vi "温度湿度监测界面.vi"() -> ()   [LabVIEW 2016, in "环境动力监测库.lvlib"]
uses:
  <vilib>/Utility/config.llb/NI_LVConfig.lvlib
  <vilib>/ptbypt/NI_PtbyPt.lvlib
panel:
  in  "湿度下限告警点":dbl
  in  "湿度上限告警点":dbl
  in  "室温下限告警点":dbl
  in  "室温上限告警点":dbl
  out "湿度":string="75.5 %"
  out "室温":string="25.8 ℃"
  # "温度湿度监测"
  # "室温:"
  # "湿度:"
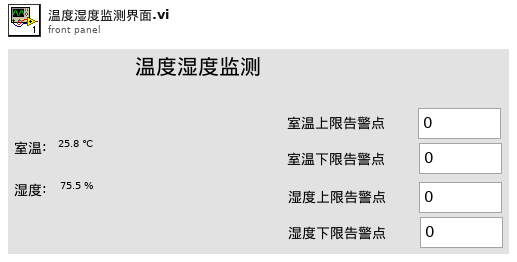
[diagram p1: front panel]
types:
  T1 = typedef "NI_LVConfig.lvlib/Config Data RefNum.ctl" = refnum<k1>
  T2 = cluster{"AD0":sgl, "AD1":sgl, "AD2":sgl, "AD3":sgl, "AD4":sgl, "AD5":sgl}
  T3 = cluster{"漏水监测配置":cluster{"监测项描述:输出":string, "端口:":enum16{"AI0", "AI1", "AI2", "AI3", "AI4", "DI0", "DI1", "DI2", "DI3", "DI4", "X0", "X1", "X2", "X3", "X4", "X5", "X6", "X7", "X8", "X9"}, "告警参数:":enum32{"禁用告警", "闭合告警", "断开告警"}, "传感器型号:":enum16{"PLC", "ZLAN"}}, "门禁开关监测配置":cluster{"监测项描述:输出":string, "端口:":enum16{"AI0", "AI1", "AI2", "AI3", "AI4", "DI0", "DI1", "DI2", "DI3", "DI4", "X0", "X1", "X2", "X3", "X4", "X5", "X6", "X7", "X8", "X9"}, "告警参数:":enum32{"禁用告警", "闭合告警", "断开告警"}, "传感器型号:":enum16{"PLC", "ZLAN"}}, "温湿度监测配置":cluster{"监测项描述:输出":string, "端口:":enum16{"AI0", "AI1", "AI2", "AI3", "AI4", "DI0", "DI1", "DI2", "DI3", "DI4", "X0", "X1", "X2", "X3", "X4", "X5", "X6", "X7", "X8", "X9"}, "告警参数:":enum32{"禁用告警", "闭合告警", "断开告警"}, "传感器型号:":enum16{"PLC", "ZLAN"}}, "烟雾监测配置":cluster{"监测项描述:输出":string, "端口:":enum16{"AI0", "AI1", "AI2", "AI3", "AI4", "DI0", "DI1", "DI2", "DI3", "DI4", "X0", "X1", "X2", "X3", "X4", "X5", "X6", "X7", "X8", "X9"}, "告警参数:":enum32{"禁用告警", "闭合告警", "断开告警"}, "传感器型号:":enum16{"PLC", "ZLAN"}}}
  T4 = cluster{"监测项描述:输出":string, "端口:":enum16{"AI0", "AI1", "AI2", "AI3", "AI4", "DI0", "DI1", "DI2", "DI3", "DI4", "X0", "X1", "X2", "X3", "X4", "X5", "X6", "X7", "X8", "X9"}, "告警参数:":enum32{"禁用告警", "闭合告警", "断开告警"}, "传感器型号:":enum16{"PLC", "ZLAN"}}
  T5 = cluster{"漏水监测输出":bool, "门禁监测输出":bool, "温湿度监测输出":bool, "烟雾监测输出":bool, "空调监测输出":bool, "自动重合闸输出":bool}
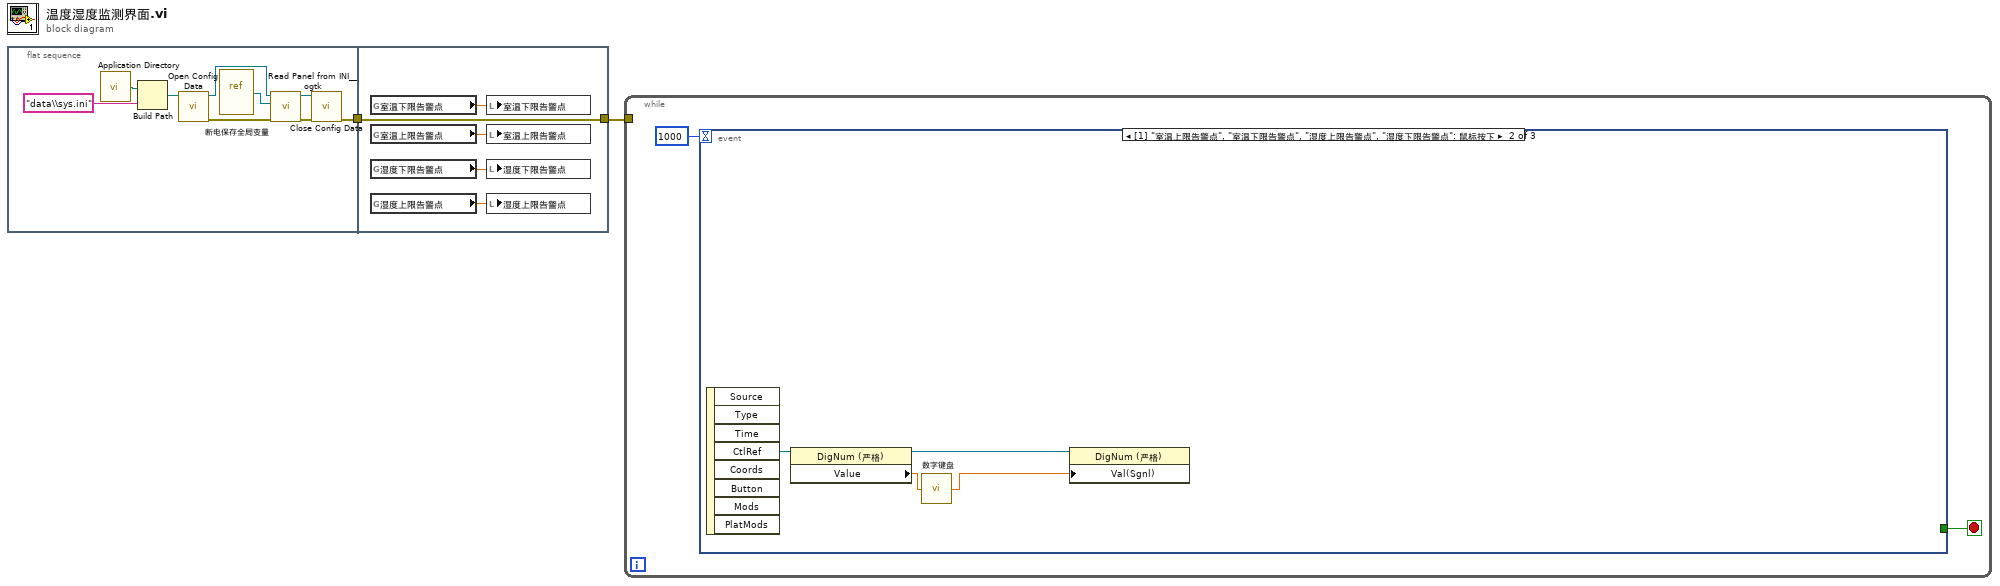
[diagram p0: block diagram]
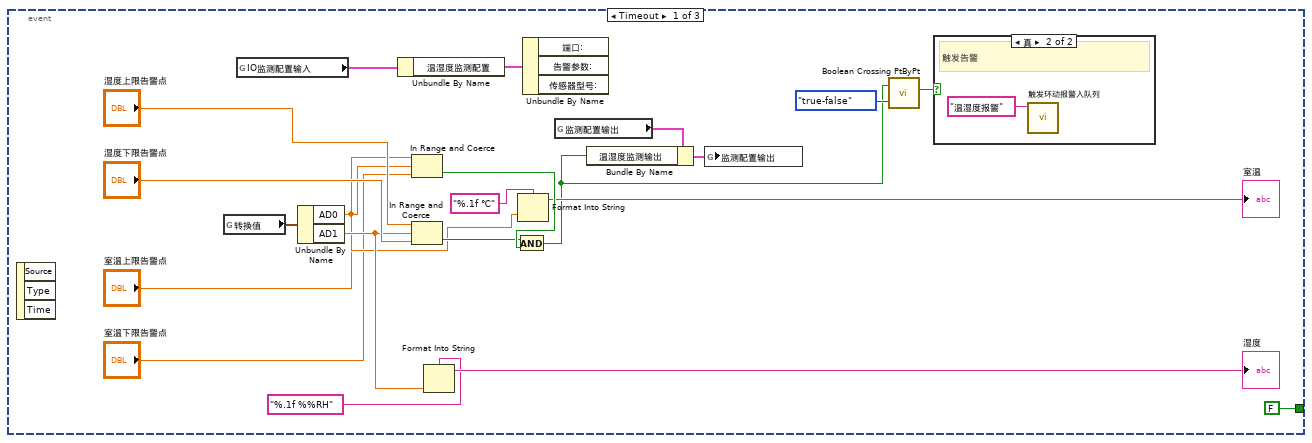
[diagram p2: hidden frame]
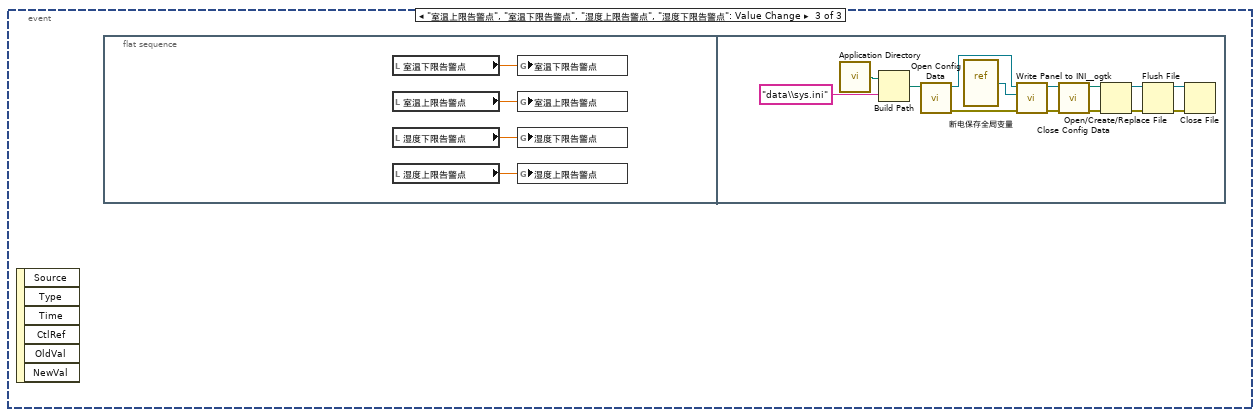
[diagram p4: hidden frame]
diagram:
  n1 = flat-sequence {
    tunnel: [w3] -> w2
    tunnel: [w16] -> w1
    tunnel: w2 -> [w16]
    frame #0 {
      n2 = call <vilib>:"Application Directory.vi"() -> ("Application Directory"=w11:path)
      n3 = Build Path(base path=w11, name or relative path="data\\sys.ini" ("名称或相对路径")) -> (appended path=w9:path)
      n4 = call <vilib>:"Open Config Data.vi"("configuration file path"=w9) -> ("error out"=w5:errorcluster, "refnum"=w8:T1)  [unwired: 8 in, 1 out]
      n5 = vi-ref "断电保存全局变量.vi"() -> (w7:refnum<vi>)
      n6 = call <userlib>:"Read Panel from INI__ogtk.vi"("error in (no error)"=w5, "VI ref"=w7, "refnum"=w8) -> ("error out"=w4:errorcluster, "refnum out"=w6:T1)  [unwired: 7 in]
      n7 = call <vilib>:"Close Config Data.vi"("error in (no error)"=w4, "refnum"=w6) -> ("error out"=w3:errorcluster)  [unwired: 8 in, 1 out]
    }
    frame #1 {
      n8 = global read "断电保存全局变量.vi" "室温下限告警点"() -> (w15:dbl)
      n9 = global read "断电保存全局变量.vi" "室温上限告警点"() -> (w14:dbl)
      n10 = global read "断电保存全局变量.vi" "湿度下限告警点"() -> (w13:dbl)
      n11 = global read "断电保存全局变量.vi" "湿度上限告警点"() -> (w12:dbl)
      n12 = local write "室温下限告警点"(w15) -> ()
      n13 = local write "室温上限告警点"(w14) -> ()
      n14 = local write "湿度下限告警点"(w13) -> ()
      n15 = local write "湿度上限告警点"(w12) -> ()
    }
  }
  n16 = while {
    tunnel: w1 -> [_]
    stop <- w18 stop-if-true
    n17 = event shown="[1] \"室温上限告警点\", \"室温下限告警点\", \"湿度上限告警点\", \"湿度下限告警点\": 鼠标按下" {
      selector: _ -> [_ _ _]
      dyn-events: _ -> [_ _ _]
      timeout: 1000 -> [_ _ _]
      tunnel: [FALSE _ _] -> w18
      event Timeout {
        n18 = event-data() -> ()  [unwired: 1 in, 3 out]
        n19 = global read "外部交互全局变量.vi" "转换值"() -> (w24:T2)
        n20 = global read "内部交互全局变量.vi" "IO监测配置输入"() -> (w27:T3)
        n21 = Unbundle By Name(w24) -> ("AD0"=w33:sgl, "AD1"=w34:sgl)
        n22 = Unbundle By Name(w27) -> ("温湿度监测配置"=w28:T4)
        n23 = In Range and Coerce(upper limit="室温上限告警点", x=w33, lower limit="室温下限告警点") -> (In Range?=w38:bool)  [unwired: 1 out]
        n24 = In Range and Coerce(upper limit="湿度上限告警点", x=w34, lower limit="湿度下限告警点") -> (In Range?=w37:bool)  [unwired: 1 out]
        n25 = Format Into String(format string="%.1f %%RH" ("格式字符串"), w34) -> (resulting string=→"湿度":string)  [unwired: 2 in, 1 out]
        n26 = And(x=w37, y=w38) -> (x .and. y?=w19:bool)
        n27 = Format Into String(format string="%.1f ℃" ("格式字符串"), w33) -> (resulting string=→"室温":string)  [unwired: 2 in, 1 out]
        n28 = Unbundle By Name(w28) -> ()  [unwired: 3 out]
        n29 = global read "内部交互全局变量.vi" "监测配置输出"() -> (w29:T5)
        n30 = Bundle By Name(cluster=w29, "温湿度监测输出"=w19) -> (w30:T5)
        n31 = global write "内部交互全局变量.vi" "监测配置输出"(w30) -> ()
        n32 = call <vilib>:"Boolean Crossing PtByPt.vi"("direction"=enum16{"either", "false-true", "true-false"}."true-false", "input"=w19) -> ("crossing"=w20:bool)  [unwired: 1 in]
        n33 = case shown="真" w20 {
          frame False {
          }
          frame True {
            # "触发告警"
            n34 = call "触发环动报警入队列.vi"("报警内容"="温湿度报警") -> ()  [unwired: 11 in]
          }
        }
      }
      event "室温上限告警点", "室温下限告警点", "湿度上限告警点", "湿度下限告警点": Mouse Down {
        n35 = event-data() -> ("CtlRef"=w44:refnum<vi>)  [unwired: 1 in, 7 out]
        n36 = property class="DigNum (严格)"(reference=w44) -> (reference out=w42:refnum<vi>, "Value"=w43:dbl)  [unwired: 1 in, 1 out]
        n37 = call "数字键盘.vi"("OldNumber"=w43) -> ("NewNumber"=w41:sgl)
        n38 = property class="DigNum (严格)"(reference=w42, "Val(Sgnl)"=w41) -> ()  [unwired: 1 in, 2 out]
      }
      event "室温上限告警点", "室温下限告警点", "湿度上限告警点", "湿度下限告警点": Value Change {
        n39 = event-data() -> ()  [unwired: 1 in, 6 out]
        n40 = flat-sequence {
          frame #0 {
            n41 = local read "室温下限告警点"() -> (w45:dbl)
            n42 = local read "室温上限告警点"() -> (w46:dbl)
            n43 = local read "湿度下限告警点"() -> (w47:dbl)
            n44 = local read "湿度上限告警点"() -> (w48:dbl)
            n45 = global write "断电保存全局变量.vi" "室温下限告警点"(w45) -> ()
            n46 = global write "断电保存全局变量.vi" "室温上限告警点"(w46) -> ()
            n47 = global write "断电保存全局变量.vi" "湿度下限告警点"(w47) -> ()
            n48 = global write "断电保存全局变量.vi" "湿度上限告警点"(w48) -> ()
          }
          frame #1 {
            n49 = call <vilib>:"Application Directory.vi"() -> ("Application Directory"=w61:path)
            n50 = Build Path(base path=w61, name or relative path="data\\sys.ini" ("名称或相对路径")) -> (appended path=w60:path)
            n51 = call <vilib>:"Open Config Data.vi"("configuration file path"=w60) -> ("error out"=w56:errorcluster, "refnum"=w59:T1)  [unwired: 8 in, 1 out]
            n52 = vi-ref "断电保存全局变量.vi"() -> (w58:refnum<vi>)
            n53 = call <userlib>:"Write Panel to INI__ogtk.vi"("error in (no error)"=w56, "VI ref"=w58, "refnum"=w59) -> ("error out"=w55:errorcluster, "refnum out"=w57:T1)  [unwired: 7 in]
            n54 = call <vilib>:"Close Config Data.vi"("error in (no error)"=w55, "refnum"=w57) -> ("error out"=w50:errorcluster, "file path"=w49:path)  [unwired: 8 in]
            n55 = Open/Create/Replace File(file path (use dialog)=w49, error in=w50) -> (refnum out=w53:refnum<file>, error out=w54:errorcluster)  [unwired: 4 in, 1 out]
            n56 = Flush File(refnum=w53, error in=w54) -> (refnum out=w52:refnum<file>, error out=w51:errorcluster)
            n57 = Close File(refnum=w52, error in=w51) -> ()  [unwired: 2 out]
          }
        }
      }
    }
  }
